vi "PS35_GetConnectInfo.vi"(3 "error in (no error)":errorcluster, 4 "Mode":i32 min=0 max=3, 5 "Control unit ID":i32=1 min=1 max=10) -> (0 "error out":errorcluster, 1 "String length":i32, 2 "Connecting info":string)   [LabVIEW 2020]
doc: "PS35_GetConnectInfo.vi, created: 03.03.2009 alex; last change: 22.10.2019 alex;\n\n<B>FUNCTION:</B> \n\nRead connecting configuration.\n----------------------------------------------------------------------------------------\n<B>INPUT:</B>\n[I32] <B>Control unit ID:</B> control unit index. (Default=1, Range=1...10) \n[I32] <B>Mode:</B> mode. (Default=0, Range=0...3) \n0 - connecting configuration\n1 - connecting configuration (short format)\n2 - last transferred data\n3 - connecting state (online or offline)\n[CLU] <B>error in</B>\n----------------------------------------------------------------------------------------\n<B>OUTPUT:</B>\n[CStr] <B>Connecting info:</B> connecting configuration or state.\n[I32] <B>String length:</B> length of the info string.\n[CLU] <B>error out</B>\n----------------------------------------------------------------------------------------\n<B>SUB-VIs:</B>\nPS35_GetReadError.vi\n----------------------------------------------------------------------------------------\n<B>EXT-Calls:</B>\nps35.dll (V2.01)\n----------------------------------------------------------------------------------------"
uses:
  ps35.dll
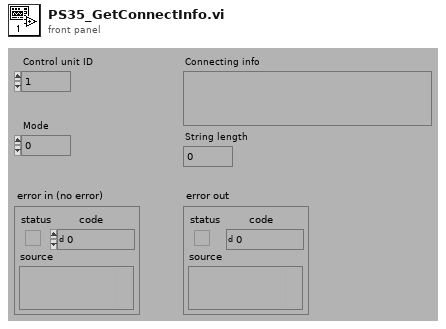
[diagram p1: front panel]
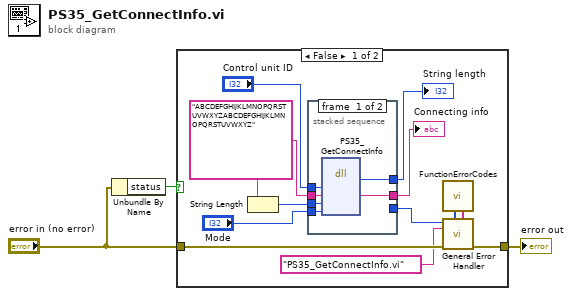
[diagram p0: block diagram]
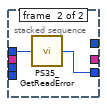
[diagram p2: hidden frame]
diagram:
  n1 = Unbundle By Name("error in (no error)") -> ("status"=w1:bool)
  n2 = case shown="False" w1 {
    tunnel: "error in (no error)" -> [w14 w24]
    tunnel: [w13 w24] -> w3
    frame False {
      w11 = "ABCDEFGHIJKLMNOPQRSTUVWXYZABCDEFGHIJKLMNOPQRSTUVWXYZ"
      n3 = String Length(string=w11) -> (length=w10:i32)
      n4 = stacked-sequence {
        tunnel: "Control unit ID" -> [w21 w23]
        tunnel: [w20 _] -> w12
        tunnel: w11 -> [w19 _]
        tunnel: w10 -> [w18 _]
        tunnel: [w17 _] -> w9
        tunnel: [_ w22] -> w8
        tunnel: "Mode" -> [w16 _]
        frame #0 {
          n5 = dll-call lib="C:/GEECS/Developers Version/source/Device Drivers/OwiSoft/OWISoftOEM/ps35/labview/lv82/ps35.dll" fn="PS35_GetConnectInfo" label="PS35_Get\nConnectInfo"("Index"=w21, "szString"=w19, "Length"=w18, "Mode"=w16) -> ("Rückgabetyp"=w17:i32, "szString"=w20:string)  [unwired: 6 in, 2 out]
        }
        frame #1 {
          n6 = call "PS35_GetReadError.vi"("Control unit ID"=w23) -> ("Read error"=w22:i32)
        }
      }
      "Connecting info" <- w12
      "String length" <- w9
      n7 = call "FunctionErrorCodes.vi"() -> ("[user-defined codes]"=w5:i32[], "[user-defined descriptions]"=w4:string[])  [unwired: 8 in]
      n8 = call <vilib>:"General Error Handler.vi"("[error code] (0)"=w8, "[user-defined codes]"=w5, "[user-defined descriptions]"=w4, "[error source] (\" \")"="PS35_GetConnectInfo.vi" ("[error source] (\" \")"), "error in (no error)"=w14) -> ("error out"=w13:errorcluster)  [unwired: 6 in, 4 out]
    }
    frame True {
    }
  }
  "error out" <- w3
